vi "Format Cors Rule.vi"(11 "Cors rule":T1) -> (3 "Cors rule string":string)   [LabVIEW 2015, in "NI_Azure_Blob.lvlib"]
uses:
  NI_Azure_Blob.lvlib
  Cors Rule.ctl
  <vilib>/Utility/error.llb/whitespace.ctl
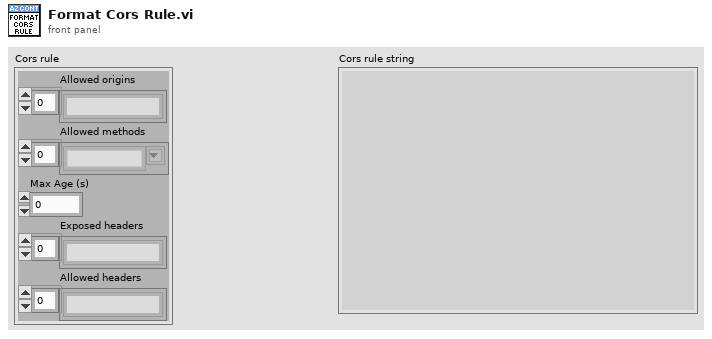
[diagram p1: front panel]
types:
  T1 = typedef "NI_Azure_Blob.lvlib/Cors Rule.ctl" = cluster{"Allowed origins":string[], "Allowed methods":string[], "Max Age (s)":u32, "Exposed headers":string[], "Allowed headers":string[]}
  T2 = typedef "whitespace.ctl" = u16
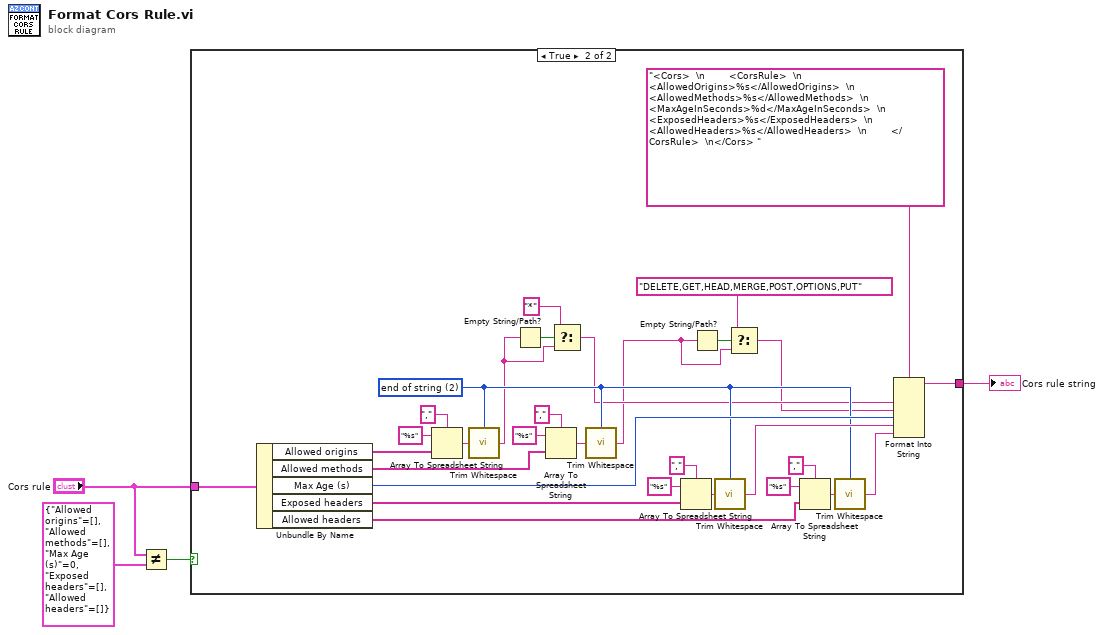
[diagram p0: block diagram]
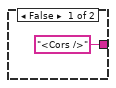
[diagram p2: hidden frame]
diagram:
  n1 = Not Equal?(x="Cors rule", y=T1 {"Allowed origins"=[], "Allowed methods"=[], "Max Age (s)"=0, "Exposed headers"=[], "Allowed headers"=[]}) -> (x != y?=w4:bool)
  n2 = case shown="True" w4 {
    tunnel: "Cors rule" -> [_ w35]
    tunnel: ["<Cors />" w34] -> w2
    frame False {
    }
    frame True {
      w14 = T2 2 items=["both", "start of string", "end of string"] ("location (both)")
      n3 = Unbundle By Name(w35) -> ("Allowed origins"=w32:string[], "Allowed methods"=w26:string[], "Max Age (s)"=w33:u32, "Exposed headers"=w23:string[], "Allowed headers"=w17:string[])
      n4 = Array To Spreadsheet String(delimiter (Tab)=",", array=w32, 3:"%s" ("format string")) -> (spreadsheet string=w29:string)
      n5 = call <vilib>:"Trim Whitespace.vi"("string"=w29, "location (both)"=w14) -> ("trimmed string"=w12:string)
      n6 = Empty String/Path?(string/path=w12) -> (empty?=w13:bool)
      n7 = Array To Spreadsheet String(delimiter (Tab)=",", array=w26, 3:"%s" ("format string")) -> (spreadsheet string=w25:string)
      n8 = Select(t="*", s=w13, f=w12) -> (s? t:f=w11:string)
      n9 = call <vilib>:"Trim Whitespace.vi"("string"=w25, "location (both)"=w14) -> ("trimmed string"=w7:string)
      n10 = Array To Spreadsheet String(delimiter (Tab)=",", array=w23, 3:"%s" ("format string")) -> (spreadsheet string=w21:string)
      n11 = Empty String/Path?(string/path=w7) -> (empty?=w8:bool)
      n12 = call <vilib>:"Trim Whitespace.vi"("string"=w21, "location (both)"=w14) -> ("trimmed string"=w16:string)
      n13 = Select(t="DELETE,GET,HEAD,MERGE,POST,OPTIONS,PUT", s=w8, f=w7) -> (s? t:f=w6:string)
      n14 = Array To Spreadsheet String(delimiter (Tab)=",", array=w17, 3:"%s" ("format string")) -> (spreadsheet string=w18:string)
      n15 = call <vilib>:"Trim Whitespace.vi"("string"=w18, "location (both)"=w14) -> ("trimmed string"=w15:string)
      n16 = Format Into String(format string="<Cors>  \n        <CorsRule>  \n            <AllowedOrigins>%s</AllowedOrigins>  \n            <AllowedMethods>%s</AllowedMethods>  \n            <MaxAgeInSeconds>%d</MaxAgeInSeconds>  \n            <ExposedHeaders>%s</ExposedHeaders>  \n            <AllowedHeaders>%s</AllowedHeaders>  \n        </CorsRule>  \n</Cors> ", w11, w6, w33, w16, w15) -> (resulting string=w34:string)  [unwired: 2 in, 1 out]
    }
  }
  "Cors rule string" <- w2
